vi "Athena Command Main.vi"() -> ()   [LabVIEW 2009]
uses:
  FPGA/FPGA Opperation Mode.ctl
  <vilib>/userDefined/High Color/nirio_resource_hc.ctl
  <vilib>/rvi/interface/nirviOpenFPGA/nirviOpenFPGA.xnode
  FPGA Bitfiles/Athena Brain.lvproj_FPGA Target 2_FPGA Main.vi.lvbitx
  <vilib>/FPGAPlugInAG/sbRIO-9642/nirviIntfOpen_sbRIO-9642.vi
  <vilib>/rvi/interface/nirviReadWriteControl/nirviReadWriteControl.xnode
  <vilib>/Utility/error.llb/Error Cluster From Error Code.vi
  <vilib>/rvi/errors/niLvFpgaAdjustHostInterfaceError.vi
  <vilib>/rvi/interface/common/niFpgaNodeNameForErrorReporting.ctl
  <vilib>/rvi/errors/niLvFpgaWhatHappensToTopLevelVI.ctl
  <vilib>/LabVIEW Targets/FPGA/RIO/nirio_HostInterface/nirio_ReadBig.vi
  <vilib>/rvi/interface/nirviCloseFPGA/nirviCloseFPGA.xnode
  <vilib>/FPGAPlugInAG/sbRIO-9642/nirviIntfClose_sbRIO-9642.vi
  NiRioSrv.dll
panel:
  in  "stop":bool
  in  "Autonomus?":bool=TRUE
  in  "Steering Position Offset":i32
  in  "Steering Control Gain":fxp<+/-,20,5>=0.149993896484375 format="%.17g"
  in  "Operation Mode":T1=enum."Autonomous"
  out "Steering Enable":bool
  out "Drive Enable":bool
  out "Speed":dbl(knob) scale=0.0..10.0
  out "Meter":i32(knob) scale=-35.0..35.0
  in  "Tab Control":enum32{"Human Control", "Autonomous"}(tab)=enum."Autonomous"
  in  "Drive Enable":bool
  in  "Steering Enable":bool
  in  "Drive Speed Current (1-3.5)":fxp<+/-,18,8> format="%.13g"
  in  "Steering Position Target":i32
  out "Drive Encoder ft/sec":fxp<+/-,18,8> format="%.13g"
  out "Drivable Paths":T2(graph)
  in  "min obstacle dist":u16=48
  in  "Autonomous Drive Current":fxp<+/-,18,8>=3.0 format="%.13g"
  out "driveable path lengths":u16[](array[numeric])
  # "Autonomous"
  # "Human Control"
  # "-35"
  # "-30"
  # "-25"
  # "-20"
  # "-15"
  # "-10"
  # "-5"
  # "-1"
  # "1"
  # "5"
  # "10"
  # "15"
  # "20"
  # "25"
  # "30"
  # "35"
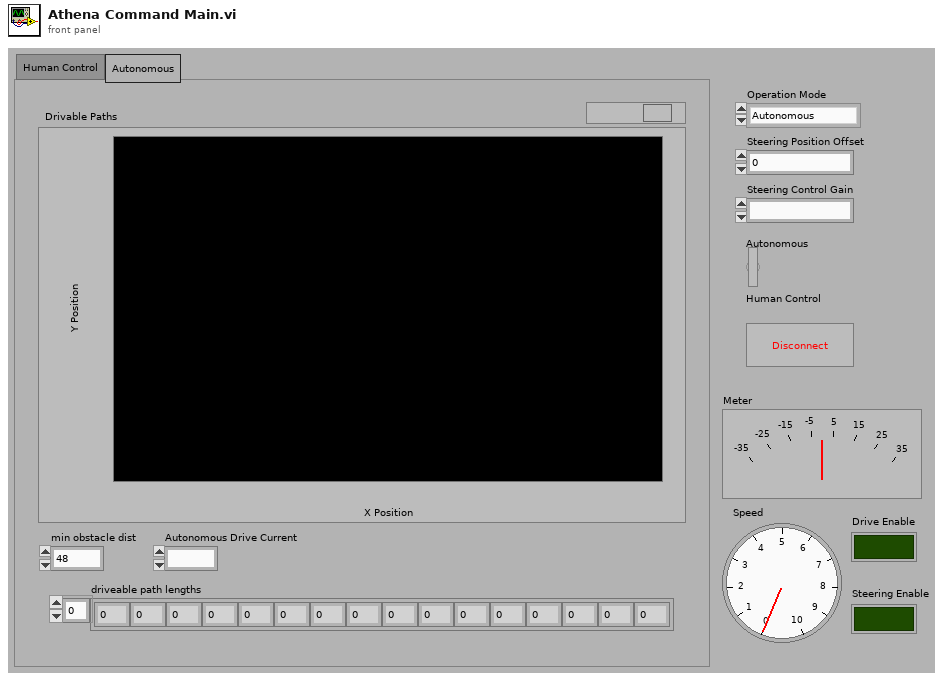
[diagram p1: front panel]
types:
  T1 = typedef "FPGA Opperation Mode.ctl" = enum16{"Human Control", "Autonomous"}
  T2 = cluster{"New X Position":i16, "New Y Position":i16}[]
  T3 = typedef "nirio_resource_hc.ctl" = tag
  T4 = typedef "niFpgaNodeNameForErrorReporting.ctl" = enum16{"Open FPGA VI Reference", "Read/Write Control", "Invoke Method: Abort", "Invoke Method: Acknowledge IRQ", "Invoke Method: Download", "Invoke Method: FIFO.Configure", "Invoke Method: FIFO.Read", "Invoke Method: FIFO.Start", "Invoke Method: FIFO.Stop", "Invoke Method: FIFO.Write", "Invoke Method: Reset", "Invoke Method: Run", "Invoke Method: Wait on IRQ", "Close FPGA VI Reference"}
  T5 = typedef "niLvFpgaWhatHappensToTopLevelVI.ctl" = enum16{"top level VI scripted behind XNode", "top level VI inlined behind XNode"}
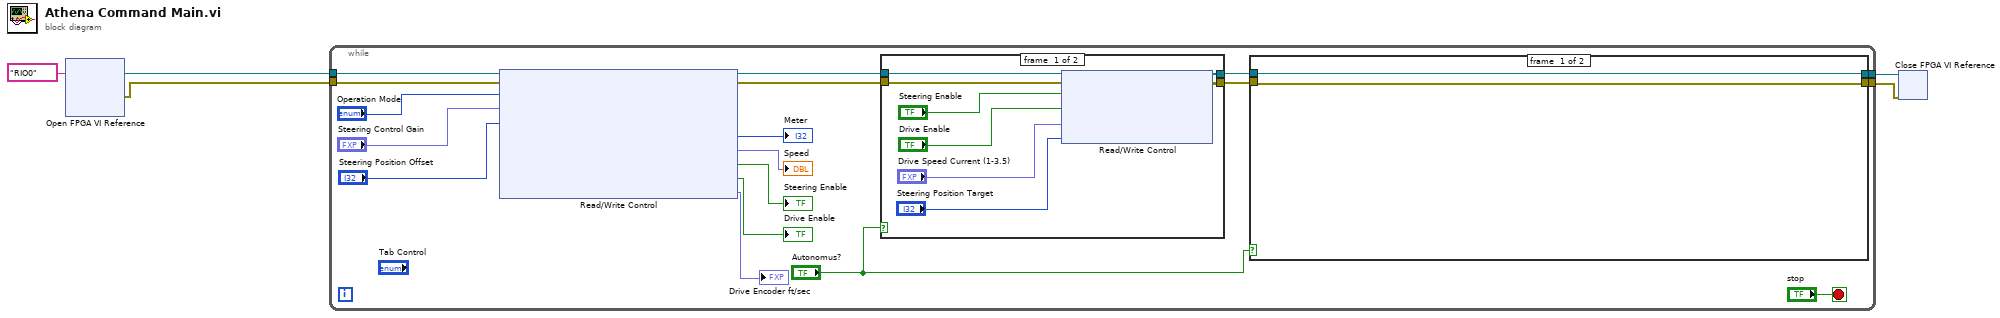
[diagram p0: block diagram]
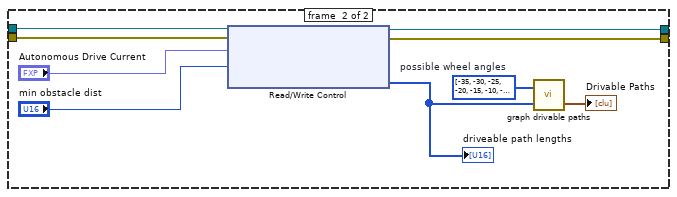
[diagram p2: hidden frame]
diagram:
  n1 = xnode "Open FPGA VI Reference"("resource name"=T3 "RIO0") -> ("FPGA VI Reference Out"=w5:refnum<k20>, "error out"=w4:errorcluster)  [unwired: 1 in]
  n2 = while {
    tunnel: w5 -> [w23]
    tunnel: w4 -> [w22]
    tunnel: [w10] -> w3
    tunnel: [w9] -> w2
    stop <- "stop" stop-if-true
    n3 = xnode "Read/Write Control"("FPGA VI Reference In"=w23, "error in"=w22, "Enum"="Operation Mode", "Steering Proportional Control Feedback Gain"="Steering Control Gain", "Steering Position Offset"="Steering Position Offset") -> ("FPGA VI Reference Out"=w21:refnum<k20>, "error out"=w20:errorcluster, "Steering Position"=→"Meter":i32, "Drive Speed Current"=→"Speed":fxp<+/-,18,8>, "Steering Enable"=→"Steering Enable":bool, "Drive Enable"=→"Drive Enable":bool, "Drive Encoder ft/sec"=→"Drive Encoder ft/sec":fxp<+/-,18,8>)
    n4 = case shown="False" "Autonomus?" {
      tunnel: w21 -> [w120 w225]
      tunnel: w20 -> [w119 w224]
      tunnel: [w114 w224] -> w19
      tunnel: [w113 w225] -> w18
      frame #0 {
        n5 = xnode "Read/Write Control"("FPGA VI Reference In"=w120, "error in"=w119, "Steering Enable"="Steering Enable", "Drive Enable"="Drive Enable", "Drive Speed Current (1-3.5)"="Drive Speed Current (1-3.5)", "Steering Position Target"="Steering Position Target") -> ("FPGA VI Reference Out"=w113:refnum<k20>, "error out"=w114:errorcluster)
      }
      frame #1 {
      }
    }
    n6 = case shown="True" "Autonomus?" {
      tunnel: w19 -> [w24 w34]
      tunnel: w18 -> [w25 w33]
      tunnel: [w25 w27] -> w10
      tunnel: [w24 w26] -> w9
      frame #0 {
      }
      frame #1 {
        w32 = i8[] [-35, -30, -25, -20, -15, -10, -5, -1, 1, 5, 10, 15, 20, 25, 30, 35]  # possible wheel angles
        n7 = xnode "Read/Write Control"("FPGA VI Reference In"=w33, "error in"=w34, "Autonomous Drive Current"="Autonomous Drive Current", "min obstacle dist"="min obstacle dist") -> ("FPGA VI Reference Out"=w27:refnum<k20>, "error out"=w26:errorcluster, "driveable path lengths"=w31:u16[])
        "driveable path lengths" <- w31
        n8 = call "graph drivable paths.vi"("updated max path lengths"=w31, "possible wheel angles"=w32) -> ("XY Graph"=→"Drivable Paths":T2)  [unwired: 1 in]
      }
    }
  }
  n9 = xnode "Close FPGA VI Reference"("FPGA VI Reference In"=w3, "error in"=w2) -> ()  [unwired: 1 out]
